vi "Add Copyright Decoration to Library.vi"() -> ()   [LabVIEW 2021, in "Utilities.lvlib"]
uses:
  Utilities.lvlib
  Error/Error.lvlib
panel:
  in  "Decoration (Partial) Content":string
  out "error out":errorcluster
  in  "Library path":path
  # "see the AlliGator License on the block diagram (Ctrl+E or Window:Show Block Diagram)"
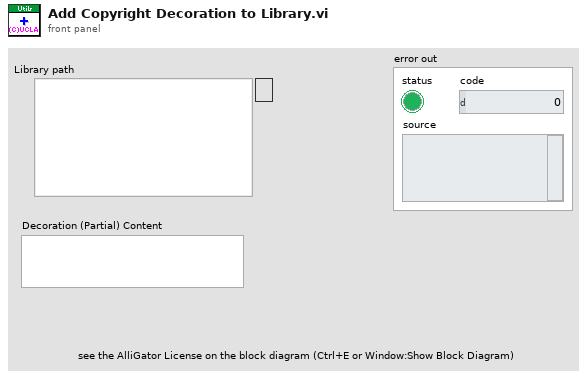
[diagram p1: front panel]
types:
  T1 = typedef "LVBoundsTypeDef.ctl" = cluster{"Width":u32, "Height":u32}
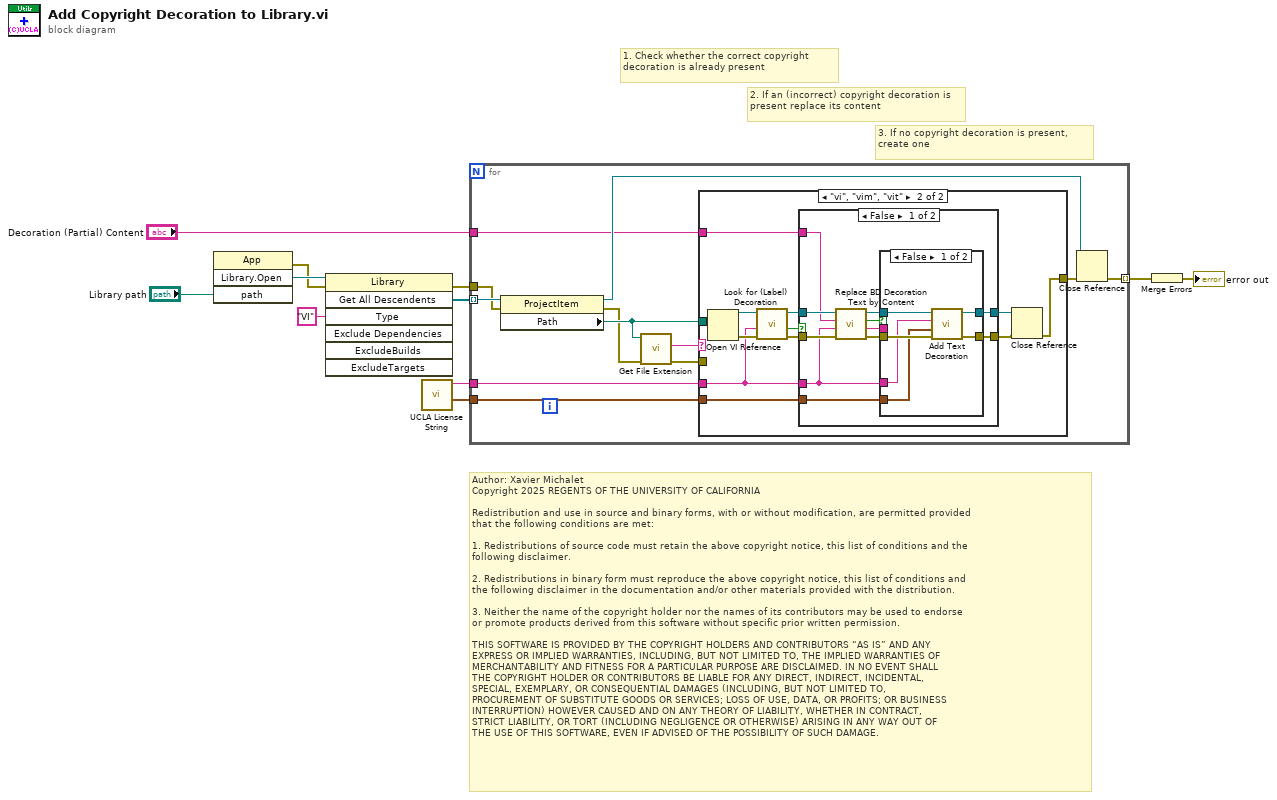
[diagram p0: block diagram]
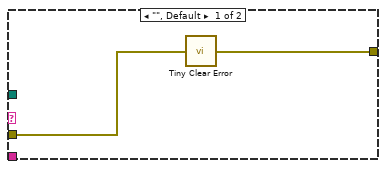
[diagram p2: hidden frame]
diagram:
  # "Author: Xavier Michalet\nCopyright 2025 REGENTS OF THE UNIVERSITY OF CALIFORNIA\n\nRedistribution and use in source and binary forms, with or without modification, are permitted provided\nthat the following conditions are met:\n\n1. Redistributions of source code must retain the above copyright notice, this list of conditions and the\nfollowing disclaimer.\n\n2. Redistributions in binary form must reproduce the above copyright notice, this list of conditions and\nthe following disclaimer in the documentation and/or other materials provided with the distribution.\n\n3. Neither the name of the copyright holder nor the names of its contributors may be used to endorse \nor promote products derived from this software without specific prior written permission.\n\nTHIS SOFTWARE IS PROVIDED BY THE COPYRIGHT HOLDERS AND CONTRIBUTORS “AS IS” AND ANY \nEXPRESS OR IMPLIED WARRANTIES, INCLUDING, BUT NOT LIMITED TO, THE IMPLIED WARRANTIES OF\nMERCHANTABILITY AND FITNESS FOR A PARTICULAR PURPOSE ARE DISCLAIMED. IN NO EVENT SHALL\nTHE COPYRIGHT HOLDER OR CONTRIBUTORS BE LIABLE FOR ANY DIRECT, INDIRECT, INCIDENTAL, \nSPECIAL, EXEMPLARY, OR CONSEQUENTIAL DAMAGES (INCLUDING, BUT NOT LIMITED TO, \nPROCUREMENT OF SUBSTITUTE GOODS OR SERVICES; LOSS OF USE, DATA, OR PROFITS; OR BUSINESS\nINTERRUPTION) HOWEVER CAUSED AND ON ANY THEORY OF LIABILITY, WHETHER IN CONTRACT, \nSTRICT LIABILITY, OR TORT (INCLUDING NEGLIGENCE OR OTHERWISE) ARISING IN ANY WAY OUT OF\nTHE USE OF THIS SOFTWARE, EVEN IF ADVISED OF THE POSSIBILITY OF SUCH DAMAGE."
  # "3. If no copyright decoration is present, create one"
  # "2. If an (incorrect) copyright decoration is present replace its content"
  # "1. Check whether the correct copyright decoration is already present"
  n1 = invoke class="App" method="Library.Open"("path"="Library path") -> (error out=w9:errorcluster, "Open Library"=w10:refnum<vi>)  [unwired: 3 in, 2 out]
  n2 = invoke class="Library" method="Get All Descendents"(reference=w10, error in=w9, "Type"="VI") -> (error out=w6:errorcluster, "All Descendents"=w7:refnum<vi>[])  [unwired: 4 in, 5 out]
  n3 = call "UCLA License String.vi"() -> ("bounds"=w3:T1, "UCLA Copyright"=w5:string)  [unwired: 10 in]
  n4 = for {
    tunnel: w7 -> [w23] mode=indexing
    tunnel: w6 -> [w22]
    tunnel: [w21] -> w2 mode=indexing
    tunnel: w5 -> [w18]
    tunnel: "Decoration (Partial) Content" -> [w17]
    tunnel: w3 -> [w16]
    n5 = property class="ProjectItem"(reference=w23, error in=w22) -> (reference out=w20:refnum<vi>, error out=w14:errorcluster, "Path"=w15:path)
    n6 = call <vilib>:"Get File Extension.vi"("error in (no error)"=w14, "file"=w15) -> ("error out"=w12:errorcluster, "lowercase file extension"=w13:string)  [unwired: 5 in, 3 out]
    n7 = case shown="\"vi\", \"vim\", \"vit\"" w13 {
      tunnel: [w24 w30] -> w19
      tunnel: w18 -> [_ w29]
      tunnel: w17 -> [_ w28]
      tunnel: w16 -> [_ w27]
      tunnel: w15 -> [_ w26]
      tunnel: w12 -> [w25 _]
      frame "", Default {
        n8 = call "Tiny Clear Error.vi"("Error In"=w25) -> ("no Error Out"=w24:errorcluster)  [unwired: 8 in]
      }
      frame "vi", "vim", "vit" {
        n9 = Open VI Reference(vi path=w26) -> (vi reference=w37:refnum<vi>, error out=w36:errorcluster)  [unwired: 5 in]
        n10 = call "Look for (Label) Decoration.vi"("error in"=w36, "Decoration Content"=w29, "VI  Ref"=w37) -> ("error out"=w34:errorcluster, "Decoration Found?"=w33:bool, "VI  Ref (dup)"=w35:refnum<vi>)  [unwired: 6 in]
        n11 = case shown="False" w33 {
          tunnel: w35 -> [w48 w58]
          tunnel: w34 -> [w47 w57]
          tunnel: [w40 w58] -> w32
          tunnel: [w44 w57] -> w31
          tunnel: w29 -> [w39 _]
          tunnel: w28 -> [w46 _]
          tunnel: w27 -> [w38 _]
          frame False {
            n12 = call "Replace BD Decoration Text by Content.vi"("error in"=w47, "New Content"=w39, "Old (partial) Content"=w46, "VI  Ref"=w48) -> ("error out"=w45:errorcluster, "Old Content"=w43:string, "VI Modified & Saved?"=w41:bool, "VI  Ref (dup)"=w42:refnum<vi>)  [unwired: 4 in]
            n13 = case shown="False" w41 {
              tunnel: w45 -> [w52 w56]
              tunnel: [w51 w56] -> w44
              tunnel: w43 -> [_ _]
              tunnel: w42 -> [w54 w55]
              tunnel: [w53 w55] -> w40
              tunnel: w39 -> [w50 _]
              tunnel: w38 -> [w49 _]
              frame False {
                n14 = call "Add Text Decoration.vi"("error in"=w52, "bounds"=w49, "Decoration Content"=w50, "VI  Ref"=w54) -> ("error out"=w51:errorcluster, "VI  Ref (dup)"=w53:refnum<vi>)  [unwired: 6 in]
              }
              frame True {
              }
            }
          }
          frame True {
          }
        }
        n15 = Close Reference(reference=w32, error in (no error)=w31) -> (error out=w30:errorcluster)
      }
    }
    n16 = Close Reference(reference=w20, error in (no error)=w19) -> (error out=w21:errorcluster)
  }
  n17 = Merge Errors(w2) -> (→"error out":errorcluster)
